vi "NInstrSim.Main_FGV.vi"() -> ()   [LabVIEW 2009, in "HB_Device_Examples.lvlib"]
doc: "Simple demo VI."
uses:
  HB_Device_Examples.lvlib
  NInstrSim/Factory/HB_DeviceFactory.lvclass
  NInstrSim/NInstrSim.lvclass
  lib.lib/HGF_LVC/HGF_BaseClasses/HGF_FGV/HGF_FGV_Clear/HGF_FGV_Clear.lvclass
  lib.lib/HGF_LVC/HGF_BaseClasses/HGF_FGV/HGF_FGV_Append/HGF_FGV_Append.lvclass
  lib.lib/HGF_LVC/HGF_BaseClasses/HGF_Factory/HGF_Factory.lvclass
  NInstrSim/Visitors/NInstrSim_ReadDCMeasurement/NInstrSim_ReadDCMeasurement.lvclass
  lib.lib/HGF_LVC/HGF_BaseClasses/HGF_FGV/HGF_FGV_Visitor/HGF_FGV_Visitor.lvclass
  NInstrSim/Visitors/NInstrSim_ReadWaveform/NInstrSim_ReadWaveform.lvclass
  NInstrSim/Visitors/NInstrSim_Visitor.lvclass
  lib.lib/HGF_LVC/HGF_BaseClasses/HGF_Notifier/HGF_Notifier.lvclass
  lib.lib/HGF_LVC/HGF_BaseClasses/HGF_FGV/HGF_FGV_Factory/HGF_FGV_Factory.lvclass
  lib.lib/HGF_LVC/HGF_Auxiliary/HGF_Auxiliary.lvlib
  lib.lib/HGF_LVC/HGF_DeviceBaseClasses/HGF_VISADevice/HGF_VISADevice.lvclass
  lib.lib/HGF_LVC/HGF_DeviceBaseClasses/HGF_DeviceBase/HGF_DeviceBase.lvclass
  HB_BaseClass_Examples.lvlib
  lib.lib/HGF_LVC/HGF_BaseClasses/HGF_FGV/HGF_FGV_VisitByName/HGF_FGV_VisitByName.lvclass
  NInstrSim/Visitors/NInstrSim_ConfigureWaveformFormat/NInstrSim_ConfigureWaveformFormat.lvclass
  NInstrSim/Visitors/NInstrSim_ConfigureWaveformType/NInstrSim_ConfigureWaveformType.lvclass
  NInstrSim/Visitors/NInstrSim_ConfigureVDCRange/NInstrSim_ConfigureVDCRange.lvclass
  lib.lib/HGF_LVC/HGF_BaseClasses/HGF_Event/HGF_Event.lvclass
panel:
  in  "timeout in ms (-1)":i32=3000
  in  "function (0:Sine)":u16(ring) items=["Sine", "Square", "Sine+Noise", "Random", "Chirp"]
  in  "Byte Order (0:Low Byte First)":u16(ring) items=["Low Byte First", "High Byte First"]
  in  "Waveform Format (0:ASCII)":u16(ring) items=["ASCII", "8-bit Unsigned Binary", "16-bit Signed Binary"]
  out "Waveform Graph":waveform(dbl)(graph)
  out "DC Measurement":dbl format="%_6g"
  in  "DC Voltage Range (1:10 VDC)":u16(ring)=1 items=["0:1 VDC", "0:10 VDC", "0:100 VDC"]
  in  "stop":bool
  out "model":string="unknown"
  out "vendor":string="unknown"
  out "firmwareRevision":string="unknown"
  out "driverRevision":string="unknown"
  out "passed?":bool
  in  "Serial Configuration":T1={"Baud Rate"=9600, "Flow Control"=0, "Parity"=0, "Data Bits"=8, "Stop Bits"=10} {"Stop Bits" items=["1.0"=10, "1.5"=15, "2.0"=20]; "Data Bits" items=["7"=7, "8"=8]; "Parity" items=["None", "Odd", "Even", "Mark", "Space"]; "Flow Control" items=["None"=0, "XON/XOFF"=1, "RTS/CTS"=2, "DTR/DSR"=4]; "Baud Rate" items=["300"=300, "600"=600, "1200"=1200, "2400"=2400, "4800"=4800, "9600"=9600, "19200"=19200]}
  in  "VISA Resource Name":refnum<visa-resource-name>
  in  "objectName":string
  out "initData found?":bool
  in  "Use Factory?":bool
  out "className":string
  out "objectName":string
  out "initialized?":bool
  out "createdFromFactory?":bool
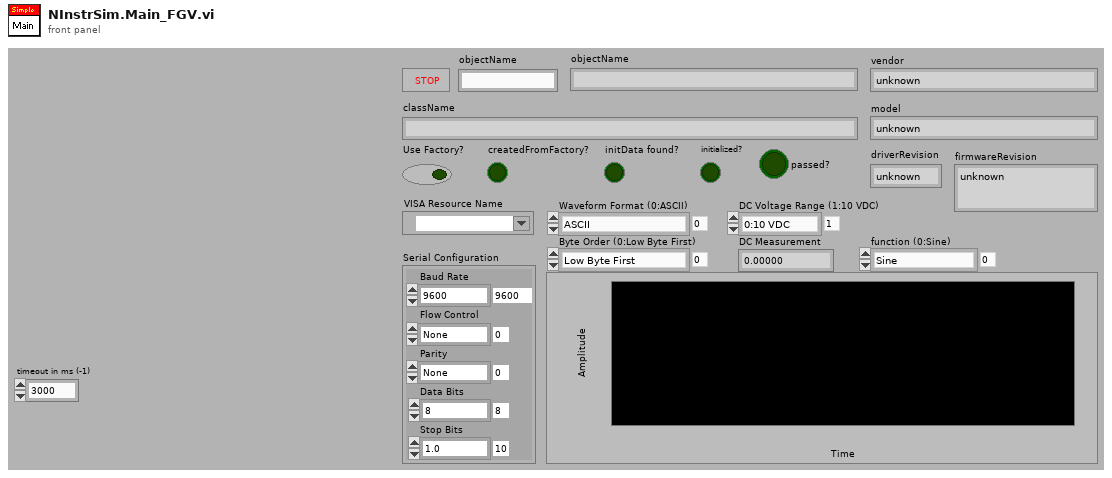
[diagram p1: front panel]
types:
  T1 = cluster{"Baud Rate":u32, "Flow Control":u16, "Parity":u16, "Data Bits":u16, "Stop Bits":u16}
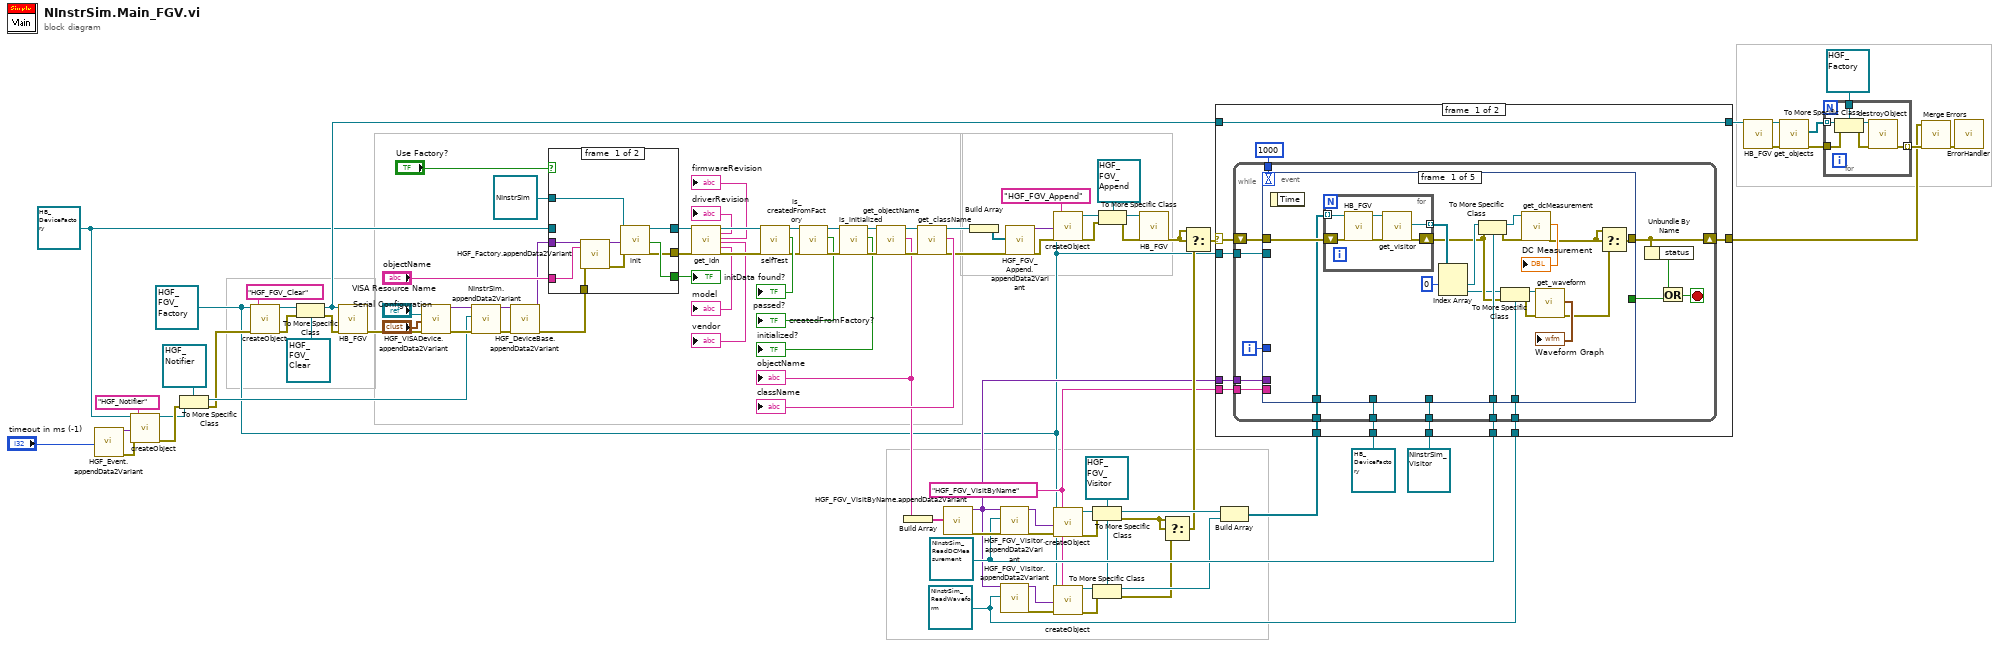
[diagram p0: block diagram]
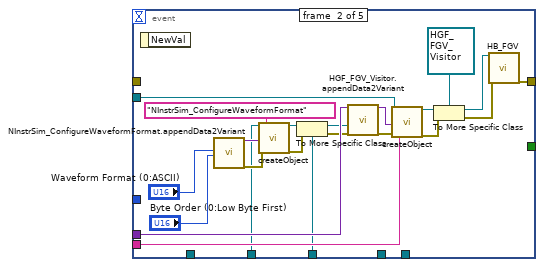
[diagram p2: hidden frame]
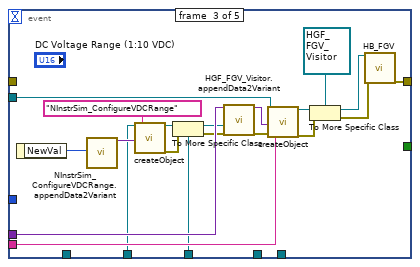
[diagram p3: hidden frame]
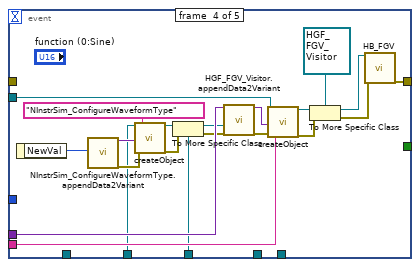
[diagram p4: hidden frame]
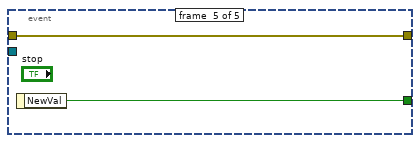
[diagram p5: hidden frame]
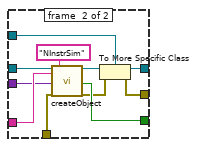
[diagram p7: hidden frame]
diagram:
  w2 = refnum<class "HGF_FGV_Factory.lvclass"> refnum ("HGF_FGV.lvlib:HGF_FGV_Factory.lvclass")
  w20 = refnum<class "NInstrSim_ReadWaveform.lvclass"> refnum ("HB_HGF_Test.lvlib:NInstrSim_ReadWaveform.lvclass")
  w27 = refnum<class "HGF_FGV_Visitor.lvclass"> refnum ("HGF_FGV.lvlib:HGF_FGV_Visitor.lvclass")
  w19 = "HGF_FGV_VisitByName" ("className")
  w37 = refnum<class "NInstrSim_ReadDCMeasurement.lvclass"> refnum ("HB_HGF_Test.lvlib:NInstrSim_ReadDCMeasurement.lvclass")
  w3 = refnum<class "HB_DeviceFactory.lvclass"> refnum ("HB_HGF_Test.lvlib:HB_Factory.lvclass")
  n1 = call "HGF_Event.appendData2Variant.vi"("timeout in ms (-1)"="timeout in ms (-1)") -> ("dup initData"=w14:variant, "error out"=w15:errorcluster)  [unwired: 2 in, 15 out]
  n2 = call "createObject.vi"("HGF_Factory"=w3, "initializationData"=w14, "error in (no error)"=w15, "className"="HGF_Notifier") -> ("HGF_Object"=w11:refnum<class "HGF_Factory.lvclass">, "error out"=w12:errorcluster)  [unwired: 2 in, 12 out]
  n3 = To More Specific Class(target class=refnum<class "HGF_Notifier.lvclass"> refnum ("HGF_BaseClasses.lvlib:HGF_Notifier.lvclass"), reference=w11, error in=w12) -> (specific class reference=w6:refnum<class "HGF_Notifier.lvclass">, error out=w4:errorcluster)
  n4 = call "createObject.vi"("HGF_Factory"=w2, "error in (no error)"=w4, "className"="HGF_FGV_Clear") -> ("HGF_Object"=w68:refnum<class "HGF_Factory.lvclass">, "error out"=w65:errorcluster)  [unwired: 2 in, 13 out]
  n5 = To More Specific Class(target class=refnum<class "HGF_FGV_Clear.lvclass"> refnum ("HGF_FGV.lvlib:HGF_FGV_Clear.lvclass"), reference=w68, error in=w65) -> (specific class reference=w34:refnum<class "HGF_FGV_Clear.lvclass">, error out=w67:errorcluster)
  n6 = call "HB_FGV.vi"("HGF_FGV_Action"=w34, "error in (no error)"=w67) -> ("error out"=w56:errorcluster)  [unwired: 17 out]
  n7 = call "HGF_VISADevice.appendData2Variant.vi"("VISA Resource Name"="VISA Resource Name", "Serial Configuration"="Serial Configuration", "error in (no error)"=w56) -> ("dup initData"=w9:variant, "error out"=w10:errorcluster)  [unwired: 1 in, 14 out]
  n8 = call "NInstrSim.appendData2Variant.vi"("initData"=w9, "statusEvent"=w6, "error in (no error)"=w10) -> ("dup initData"=w8:variant, "error out"=w7:errorcluster)  [unwired: 15 out]
  n9 = call "HGF_DeviceBase.appendData2Variant.vi"("initData"=w8, "error in (no error)"=w7) -> ("dup initData"=w84:variant, "error out"=w83:errorcluster)  [unwired: 16 out]
  n10 = case shown="True" "Use Factory?" {
    tunnel: [w105 w114] -> w80
    tunnel: [w103 w111] -> w79
    tunnel: refnum<class "NInstrSim.lvclass"> refnum ("HB_HGF_Test.lvlib:NInstrSim.lvclass") -> [w100 w112]
    tunnel: [w104 w115] -> w87
    tunnel: w3 -> [_ w110]
    tunnel: "objectName" -> [w97 w109]
    tunnel: w84 -> [w99 w107]
    tunnel: w83 -> [w98 w106]
    frame #0 {
      n11 = call "HGF_Factory.appendData2Variant.vi"("initData"=w99, "objectName"=w97, "error in (no error)"=w98) -> ("dup initData"=w101:variant, "error out"=w102:errorcluster)  [unwired: 2 in, 13 out]
      n12 = call "init.vi"("HGF_Object"=w100, "initializationData"=w101, "error in (no error)"=w102) -> ("dup HGF_Object"=w105:refnum<class "NInstrSim.lvclass">, "found?"=w104:bool, "error out"=w103:errorcluster)  [unwired: 14 out]
    }
    frame #1 {
      n13 = call "createObject.vi"("HGF_Factory"=w110, "objectName"=w109, "initializationData"=w107, "error in (no error)"=w106, "className"="NInstrSim") -> ("HGF_Object"=w108:refnum<class "HGF_Factory.lvclass">, "found?"=w115:bool, "error out"=w113:errorcluster)  [unwired: 12 out]
      n14 = To More Specific Class(target class=w112, reference=w108, error in=w113) -> (specific class reference=w114:refnum<class "NInstrSim.lvclass">, error out=w111:errorcluster)
    }
  }
  "initData found?" <- w87
  n15 = call "get_idn.vi"("HGF_DeviceBase"=w80, "error in (no error)"=w79) -> ("dup HGF_DeviceBase"=w78:refnum<class "NInstrSim.lvclass">, "driverRevision"=→"driverRevision":string, "firmwareRevision"=→"firmwareRevision":string, "vendor"=→"vendor":string, "model"=→"model":string, "error out"=w77:errorcluster)  [unwired: 12 out]
  n16 = call-dynamic "selfTest.vi"("NInstrSim"=w78, "error in (no error)"=w77) -> ("dup NInstrSim"=w71:refnum<class "NInstrSim.lvclass">, "passed?"=→"passed?":bool, "error out"=w70:errorcluster)  [unwired: 15 out]
  n17 = call "is_createdFromFactory.vi"("HGF_Factory"=w71, "error in (no error)"=w70) -> ("dup HGF_Factory"=w69:refnum<class "NInstrSim.lvclass">, "createdFromFactory?"=→"createdFromFactory?":bool, "error out"=w96:errorcluster)  [unwired: 15 out]
  n18 = call "is_initialized.vi"("HGF_Factory"=w69, "error in (no error)"=w96) -> ("dup HGF_Factory"=w95:refnum<class "NInstrSim.lvclass">, "initialized?"=→"initialized?":bool, "error out"=w94:errorcluster)  [unwired: 15 out]
  n19 = call "get_objectName.vi"("HGF_Factory"=w95, "error in (no error)"=w94) -> ("dup HGF_Factory"=w91:refnum<class "NInstrSim.lvclass">, "objectName"=w44:string, "error out"=w90:errorcluster)  [unwired: 15 out]
  "objectName" <- w44
  n20 = Build Array(w44) -> (w43:string[])
  n21 = call "get_className.vi"("HGF_Factory"=w91, "error in (no error)"=w90) -> ("dup HGF_Factory"=w54:refnum<class "NInstrSim.lvclass">, "className"=→"className":string, "error out"=w52:errorcluster)  [unwired: 15 out]
  n22 = call "HGF_FGV_VisitByName.appendData2Variant.vi"("nameArray"=w43) -> ("dup initData"=w18:variant, "error out"=w42:errorcluster)  [unwired: 2 in, 15 out]
  n23 = Build Array(w54) -> (w55:refnum<class "NInstrSim.lvclass">[])
  n24 = call "HGF_FGV_Visitor.appendData2Variant.vi"("initData"=w18, "HGF_Visitor"=w37, "error in (no error)"=w42) -> ("dup initData"=w41:variant, "error out"=w40:errorcluster)  [unwired: 15 out]
  n25 = call "HGF_FGV_Visitor.appendData2Variant.vi"("initData"=w18, "HGF_Visitor"=w20) -> ("dup initData"=w28:variant, "error out"=w29:errorcluster)  [unwired: 1 in, 15 out]
  n26 = call "HGF_FGV_Append.appendData2Variant.vi"("Objects"=w55, "error in (no error)"=w52) -> ("dup initData"=w57:variant, "error out"=w53:errorcluster)  [unwired: 1 in, 15 out]
  n27 = call "createObject.vi"("HGF_Factory"=w2, "initializationData"=w57, "error in (no error)"=w53, "className"="HGF_FGV_Append") -> ("HGF_Object"=w63:refnum<class "HGF_Factory.lvclass">, "error out"=w60:errorcluster)  [unwired: 1 in, 13 out]
  n28 = call "createObject.vi"("HGF_Factory"=w2, "initializationData"=w41, "error in (no error)"=w40, "className"=w19) -> ("HGF_Object"=w39:refnum<class "HGF_Factory.lvclass">, "error out"=w38:errorcluster)  [unwired: 1 in, 13 out]
  n29 = call "createObject.vi"("HGF_Factory"=w2, "initializationData"=w28, "error in (no error)"=w29, "className"=w19) -> ("HGF_Object"=w30:refnum<class "HGF_Factory.lvclass">, "error out"=w31:errorcluster)  [unwired: 1 in, 13 out]
  n30 = To More Specific Class(target class=w27, reference=w39, error in=w38) -> (specific class reference=w26:refnum<class "HGF_FGV_Visitor.lvclass">, error out=w23:errorcluster)
  n31 = To More Specific Class(target class=w27, reference=w30, error in=w31) -> (specific class reference=w24:refnum<class "HGF_FGV_Visitor.lvclass">, error out=w21:errorcluster)
  n32 = To More Specific Class(target class=refnum<class "HGF_FGV_Append.lvclass"> refnum ("HGF_FGV.lvlib:HGF_FGV_Append.lvclass"), reference=w63, error in=w60) -> (specific class reference=w61:refnum<class "HGF_FGV_Append.lvclass">, error out=w62:errorcluster)
  n33 = call "HB_FGV.vi"("HGF_FGV_Action"=w61, "error in (no error)"=w62) -> ("error out"=w36:errorcluster)  [unwired: 17 out]
  n34 = Select(t=w23, s=w23, f=w21) -> (s? t:f=w22:errorcluster)
  n35 = Select(t=w36, s=w36, f=w22) -> (s? t:f=w35:errorcluster)
  n36 = Build Array(w26, w24) -> (w25:refnum<class "HGF_FGV_Visitor.lvclass">[])
  n37 = case shown="No Error" w35 {
    selector: w35 -> [w128 w234]
    tunnel: [w127 w234] -> w32
    tunnel: w25 -> [w125 _]
    tunnel: w37 -> [w124 _]
    tunnel: w34 -> [w123 w233]
    tunnel: [w123 w233] -> w33
    tunnel: w20 -> [w122 _]
    tunnel: w19 -> [w121 _]
    tunnel: w18 -> [w120 _]
    tunnel: refnum<class "NInstrSim_Visitor.lvclass"> refnum ("HB_HGF_Test.lvlib:NInstrSim_Visitor.lvclass") -> [w119 _]
    tunnel: w2 -> [w118 _]
    tunnel: refnum<class "HB_DeviceFactory.lvclass"> refnum ("HB_HGF_Test.lvlib:HB_Factory.lvclass") -> [w117 _]
    frame #0 {
      n38 = while {
        shift-right: [w140] -> w127
        shift-left: w128 -> [w143]
        tunnel: 1000 -> [w138]
        tunnel: w125 -> [w136]
        tunnel: w124 -> [w135]
        tunnel: w122 -> [w134]
        tunnel: w121 -> [w133]
        tunnel: w120 -> [w132]
        tunnel: w119 -> [w131]
        tunnel: w118 -> [w130]
        tunnel: w117 -> [w129]
        i -> [w137]
        stop <- w141 stop-if-true
        n39 = event shown="[1] \"Waveform Format (0:ASCII)\", \"Byte Order (0:Low Byte First)\": Value Change" {
          selector: _ -> [_ _ _ _ _]
          dyn-events: _ -> [_ _ _ _ _]
          timeout: w138 -> [_ _ _ _ _]
          tunnel: w143 -> [w161 _ _ _ w232]
          tunnel: [w146 w184 w204 w225 w232] -> w140
          tunnel: [_ _ _ _ w231] -> w142
          tunnel: w137 -> [_ _ _ _ _]
          tunnel: w136 -> [w160 _ _ _ _]
          tunnel: w135 -> [w158 _ _ _ _]
          tunnel: w134 -> [w151 _ _ _ _]
          tunnel: w133 -> [_ w185 w205 w226 _]
          tunnel: w132 -> [_ w181 w201 w222 _]
          tunnel: w131 -> [_ w179 w199 w220 _]
          tunnel: w130 -> [_ w173 w194 w215 _]
          tunnel: w129 -> [_ w168 w190 w210 _]
          event #0 {
            n40 = event-data() -> ()  [unwired: 2 out]
            n41 = for {
              tunnel: w160 -> [w166] mode=indexing
              tunnel: [w163] -> w154 mode=indexing
              shift-right: [w162] -> w152
              shift-left: w161 -> [w167]
              n42 = call "HB_FGV.vi"("HGF_FGV_Action"=w166, "error in (no error)"=w167) -> ("dup HGF_FGV_Action"=w165:refnum<class "HGF_FGV_Visitor.lvclass">, "error out"=w164:errorcluster)  [unwired: 16 out]
              n43 = call "get_visitor.vi"("HGF_FGV_Visitor"=w165, "error in (no error)"=w164) -> ("visitor"=w163:refnum<class "HGF_Visitor.lvclass">, "error out"=w162:errorcluster)  [unwired: 16 out]
            }
            n44 = Index Array(array=w154, index #1=0 ("index")) -> (element #1=w155:refnum<class "HGF_Visitor.lvclass">, element #2=w150:refnum<class "HGF_Visitor.lvclass">)  [unwired: 1 in]
            n45 = To More Specific Class(target class=w158, reference=w155, error in=w152) -> (specific class reference=w157:refnum<class "NInstrSim_ReadDCMeasurement.lvclass">, error out=w159:errorcluster)
            n46 = To More Specific Class(target class=w151, reference=w150, error in=w152) -> (specific class reference=w149:refnum<class "NInstrSim_ReadWaveform.lvclass">, error out=w148:errorcluster)
            n47 = call "get_dcMeasurement.vi"("NInstrSim_ReadDCMeasurement"=w157, "error in (no error)"=w159) -> ("dcMeasurement"=→"DC Measurement":dbl, "error out"=w145:errorcluster)  [unwired: 16 out]
            n48 = call "get_waveform.vi"("NInstrSim_ReadWaveform"=w149, "error in (no error)"=w148) -> ("Waveform"=→"Waveform Graph":waveform(dbl), "error out"=w144:errorcluster)  [unwired: 16 out]
            n49 = Select(t=w145, s=w145, f=w144) -> (s? t:f=w146:errorcluster)
          }
          event #1 {
            n50 = event-data() -> ()  [unwired: 2 out]
            n51 = call "NInstrSim_ConfigureWaveformFormat.appendData2Variant.vi"("format (0:ASCII)"="Waveform Format (0:ASCII)", "byteOrder (0:Low Byte First)"="Byte Order (0:Low Byte First)") -> ("dup initData"=w176:variant, "error out"=w170:errorcluster)  [unwired: 2 in, 14 out]
            n52 = call "createObject.vi"("HGF_Factory"=w168, "initializationData"=w176, "error in (no error)"=w170, "className"="NInstrSim_ConfigureWaveformFormat") -> ("HGF_Object"=w177:refnum<class "HGF_Factory.lvclass">, "error out"=w171:errorcluster)  [unwired: 1 in, 13 out]
            n53 = To More Specific Class(target class=w179, reference=w177, error in=w171) -> (specific class reference=w172:refnum<class "NInstrSim_Visitor.lvclass">, error out=w180:errorcluster)
            n54 = call "HGF_FGV_Visitor.appendData2Variant.vi"("initData"=w181, "HGF_Visitor"=w172, "error in (no error)"=w180) -> ("dup initData"=w186:variant, "error out"=w187:errorcluster)  [unwired: 15 out]
            n55 = call "createObject.vi"("HGF_Factory"=w173, "initializationData"=w186, "error in (no error)"=w187, "className"=w185) -> ("HGF_Object"=w188:refnum<class "HGF_Factory.lvclass">, "error out"=w189:errorcluster)  [unwired: 1 in, 13 out]
            n56 = To More Specific Class(target class=refnum<class "HGF_FGV_Visitor.lvclass"> refnum ("HGF_FGV.lvlib:HGF_FGV_Visitor.lvclass"), reference=w188, error in=w189) -> (specific class reference=w182:refnum<class "HGF_FGV_Visitor.lvclass">, error out=w169:errorcluster)
            n57 = call "HB_FGV.vi"("HGF_FGV_Action"=w182, "error in (no error)"=w169) -> ("error out"=w184:errorcluster)  [unwired: 17 out]
          }
          event #2 {
            n58 = event-data() -> ("NewVal"=w195:u16)  [unwired: 1 out]
            n59 = call "NInstrSim_ConfigureVDCRange.appendData2Variant.vi"("DC Voltage Range (1:10 VDC)"=w195) -> ("dup initData"=w196:variant)  [unwired: 2 in, 16 out]
            n60 = call "createObject.vi"("HGF_Factory"=w190, "initializationData"=w196, "className"="NInstrSim_ConfigureVDCRange") -> ("HGF_Object"=w197:refnum<class "HGF_Factory.lvclass">, "error out"=w192:errorcluster)  [unwired: 2 in, 13 out]
            n61 = To More Specific Class(target class=w199, reference=w197, error in=w192) -> (specific class reference=w193:refnum<class "NInstrSim_Visitor.lvclass">, error out=w200:errorcluster)
            n62 = call "HGF_FGV_Visitor.appendData2Variant.vi"("initData"=w201, "HGF_Visitor"=w193, "error in (no error)"=w200) -> ("dup initData"=w206:variant, "error out"=w207:errorcluster)  [unwired: 15 out]
            n63 = call "createObject.vi"("HGF_Factory"=w194, "initializationData"=w206, "error in (no error)"=w207, "className"=w205) -> ("HGF_Object"=w208:refnum<class "HGF_Factory.lvclass">, "error out"=w209:errorcluster)  [unwired: 1 in, 13 out]
            n64 = To More Specific Class(target class=refnum<class "HGF_FGV_Visitor.lvclass"> refnum ("HGF_FGV.lvlib:HGF_FGV_Visitor.lvclass"), reference=w208, error in=w209) -> (specific class reference=w202:refnum<class "HGF_FGV_Visitor.lvclass">, error out=w191:errorcluster)
            n65 = call "HB_FGV.vi"("HGF_FGV_Action"=w202, "error in (no error)"=w191) -> ("error out"=w204:errorcluster)  [unwired: 17 out]
          }
          event #3 {
            n66 = event-data() -> ("NewVal"=w217:u16)  [unwired: 1 out]
            n67 = call "NInstrSim_ConfigureWaveformType.appendData2Variant.vi"("function (0:Sine)"=w217) -> ("dup initData"=w216:variant, "error out"=w211:errorcluster)  [unwired: 2 in, 15 out]
            n68 = call "createObject.vi"("HGF_Factory"=w210, "initializationData"=w216, "error in (no error)"=w211, "className"="NInstrSim_ConfigureWaveformType") -> ("HGF_Object"=w218:refnum<class "HGF_Factory.lvclass">, "error out"=w213:errorcluster)  [unwired: 1 in, 13 out]
            n69 = To More Specific Class(target class=w220, reference=w218, error in=w213) -> (specific class reference=w214:refnum<class "NInstrSim_Visitor.lvclass">, error out=w221:errorcluster)
            n70 = call "HGF_FGV_Visitor.appendData2Variant.vi"("initData"=w222, "HGF_Visitor"=w214, "error in (no error)"=w221) -> ("dup initData"=w227:variant, "error out"=w228:errorcluster)  [unwired: 15 out]
            n71 = call "createObject.vi"("HGF_Factory"=w215, "initializationData"=w227, "error in (no error)"=w228, "className"=w226) -> ("HGF_Object"=w229:refnum<class "HGF_Factory.lvclass">, "error out"=w230:errorcluster)  [unwired: 1 in, 13 out]
            n72 = To More Specific Class(target class=refnum<class "HGF_FGV_Visitor.lvclass"> refnum ("HGF_FGV.lvlib:HGF_FGV_Visitor.lvclass"), reference=w229, error in=w230) -> (specific class reference=w223:refnum<class "HGF_FGV_Visitor.lvclass">, error out=w212:errorcluster)
            n73 = call "HB_FGV.vi"("HGF_FGV_Action"=w223, "error in (no error)"=w212) -> ("error out"=w225:errorcluster)  [unwired: 17 out]
          }
          event #4 {
            n74 = event-data() -> ("NewVal"=w231:bool)  [unwired: 1 out]
          }
        }
        n75 = Unbundle By Name(w140) -> ("status"=w139:bool)
        n76 = Or(x=w139, y=w142) -> (x .or. y?=w141:bool)
      }
    }
    frame #1 {
    }
  }
  n77 = call "HB_FGV.vi"("HGF_FGV_Action"=w33) -> ("dup HGF_FGV_Action"=w50:refnum<class "HGF_FGV_Clear.lvclass">, "error out"=w51:errorcluster)  [unwired: 1 in, 16 out]
  n78 = call "get_objects.vi"("HGF_FGV_Clear"=w50, "error in (no error)"=w51) -> ("objects"=w49:refnum<class>[], "error out"=w48:errorcluster)  [unwired: 16 out]
  n79 = for {
    tunnel: [w240] -> w47 mode=indexing
    tunnel: w49 -> [w239] mode=indexing
    tunnel: w48 -> [w238]
    tunnel: refnum<class "HGF_Factory.lvclass"> refnum ("HGF_BaseClasses.lvlib:HGF_Factory.lvclass") -> [w235]
    n80 = To More Specific Class(target class=w235, reference=w239, error in=w238) -> (specific class reference=w236:refnum<class "HGF_Factory.lvclass">, error out=w237:errorcluster)
    n81 = call "destroyObject.vi"("HGF_Factory"=w236, "error in (no error)"=w237) -> ("error out"=w240:errorcluster)  [unwired: 17 out]
  }
  n82 = call <vilib>:"Merge Errors.vi"("error array in"=w47, "error in 1 (no error)"=w32) -> ("error out"=w46:errorcluster)  [unwired: 2 in, 3 out]
  n83 = call "ErrorHandler.vi"("error in (no error)"=w46) -> ()  [unwired: 6 in, 13 out]
